vi "Test.vi"() -> ()   [LabVIEW 2017]
uses:
  Controls/saveDataOption.ctl
  TypeDefs/Trav-Command-TD.ctl
  Globals/measurementGlobal.vi
  <vilib>/Utility/file.llb/Read Delimited Spreadsheet (I64).vi
panel:
  in  "Boolean":bool
  in  "Trav Command":T1 items=["Set Reference", "Read Position", "Move", "StopMotors"]
  out "Traverse Position":i32[][](array[numeric])
  out "Block Index":i32
  in  "Setup":enum16{"Run Programme", "Show Setup"}(ring)
  in  "Data Acquisition":T2(ring)
  in  "Save Data Option":T3
  in  "Tap Control":enum32{"Plots", "Status and File"}(tab)
  out "Waveform Graph":dbl[](graph)
  out "Waveform Chart":dbl[][](graph)
  in  "Folder Path":path
  out "Comments":string
  # "ON"
  # "OFF"
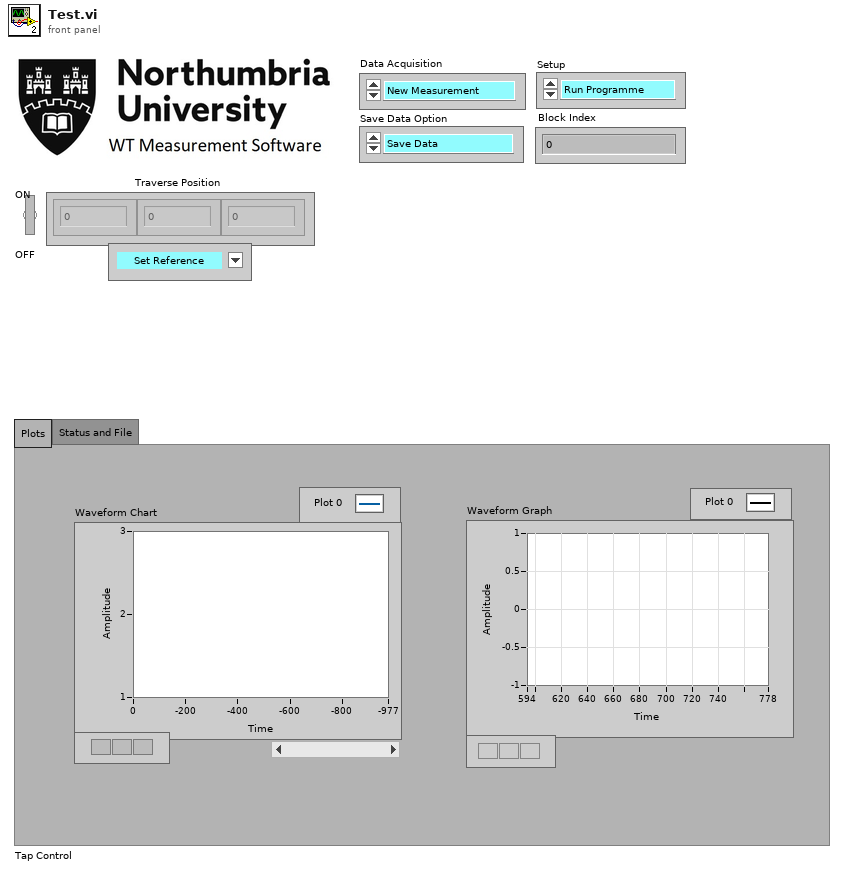
[diagram p1: front panel]
types:
  T1 = typedef "Trav-Command-TD.ctl" = u16
  T2 = enum16{"New Measurement", "Post-process Raw Data"}
  T3 = typedef "saveDataOption.ctl" = enum16{"Save Data", "Do Not Save Data"}
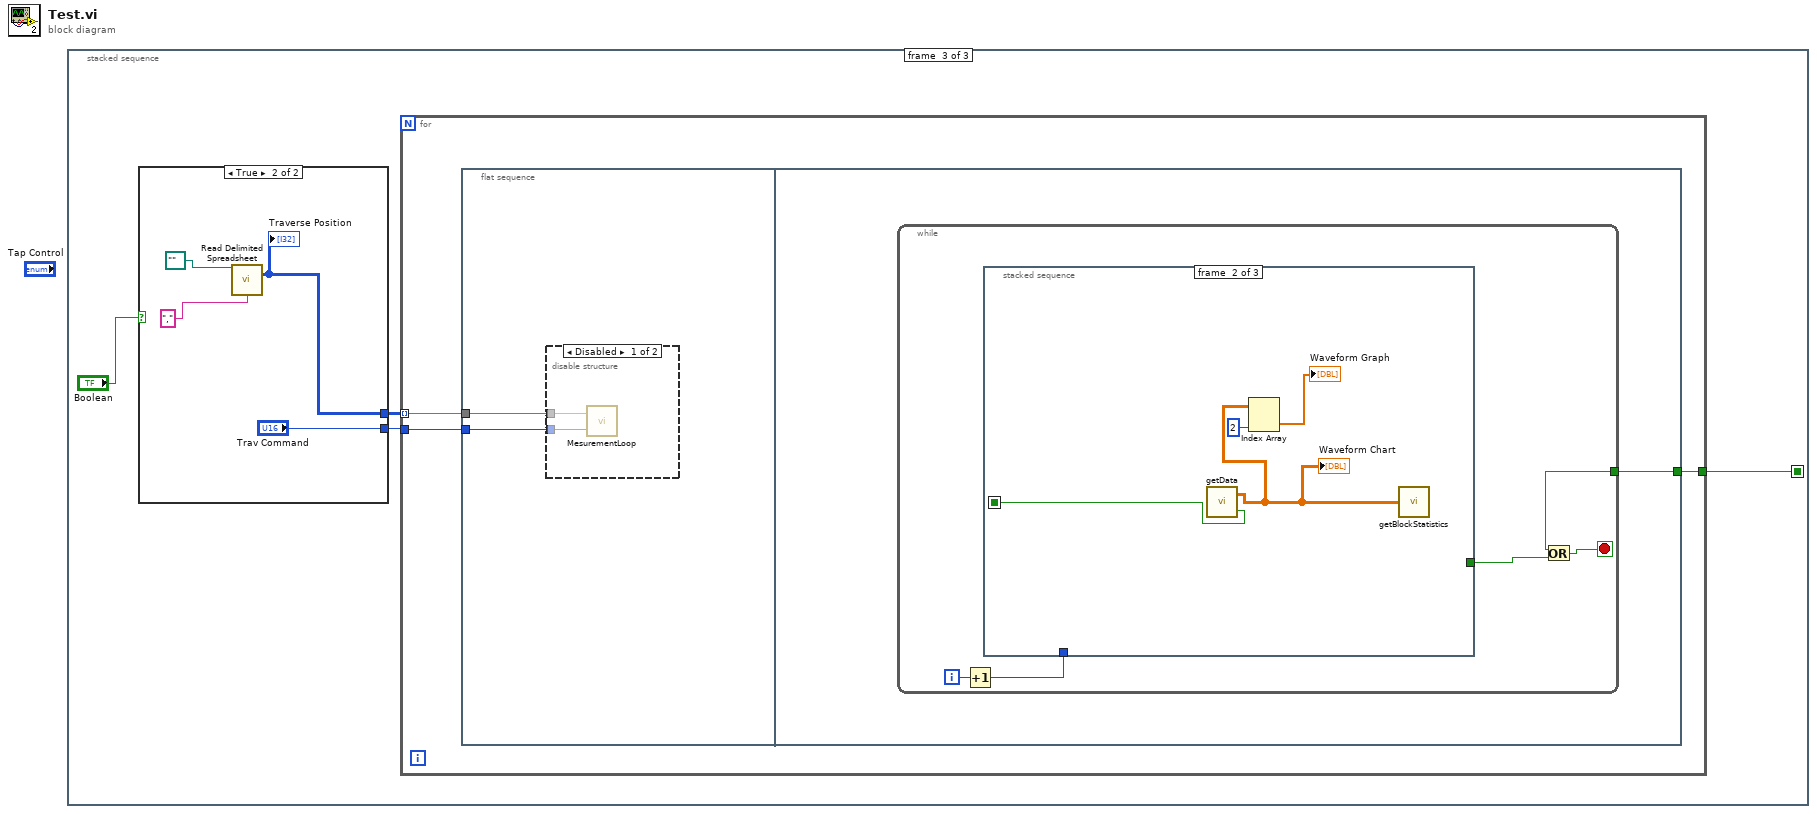
[diagram p0: block diagram]
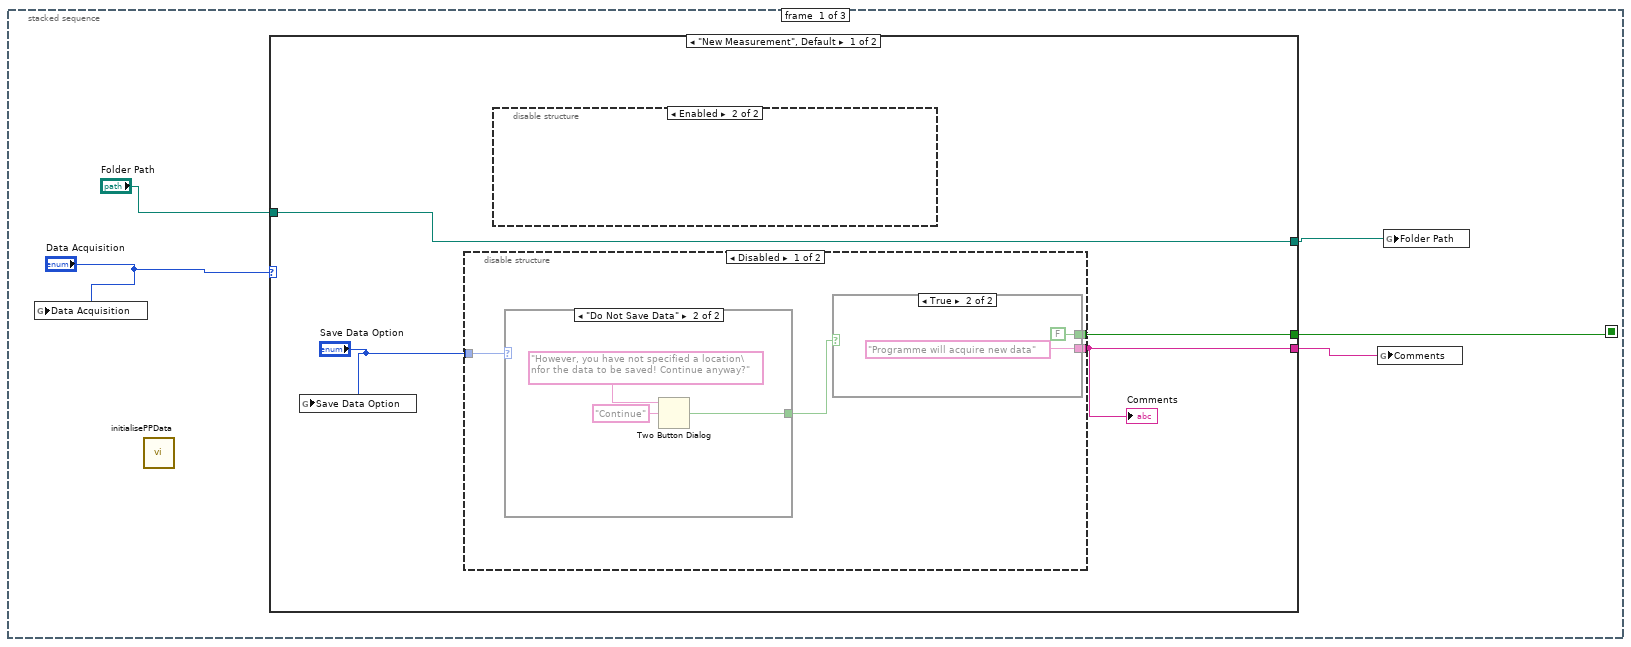
[diagram p2: hidden frame]
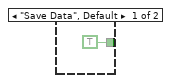
[diagram p3: hidden frame]
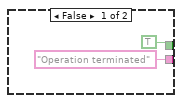
[diagram p4: hidden frame]
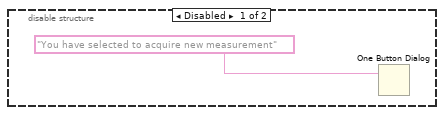
[diagram p6: hidden frame]
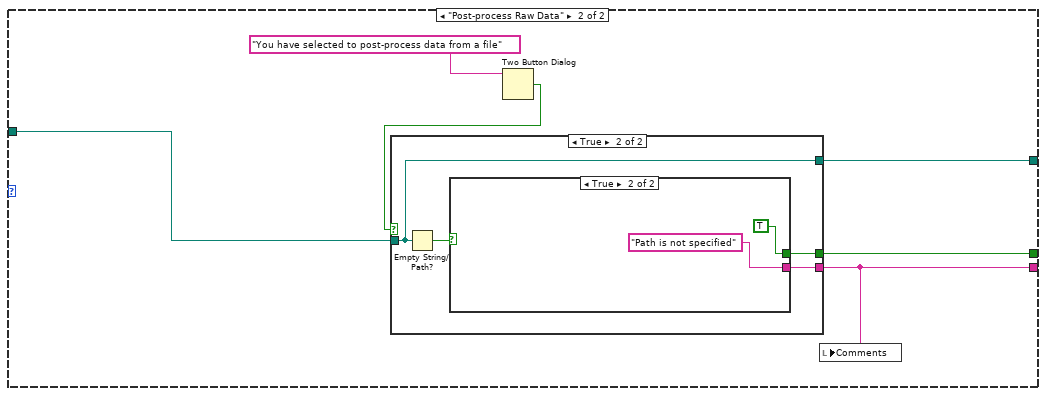
[diagram p7: hidden frame]
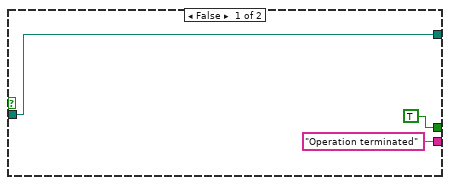
[diagram p8: hidden frame]
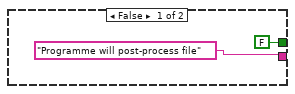
[diagram p9: hidden frame]
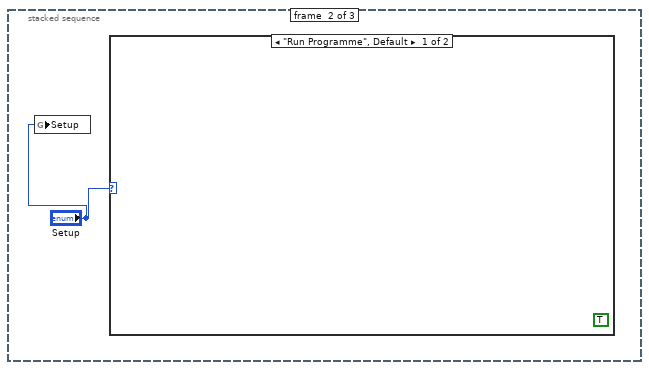
[diagram p10: hidden frame]
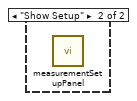
[diagram p11: hidden frame]
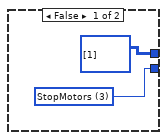
[diagram p12: hidden frame]
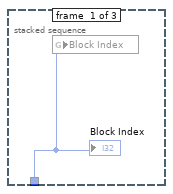
[diagram p14: hidden frame]
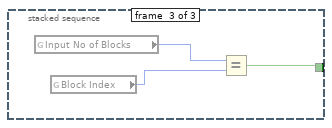
[diagram p15: hidden frame]
diagram:
  n1 = stacked-sequence {
    seq-local: [w3 _ _] -> [_ _ w44]
    frame #0 {
      n2 = global write "measurementGlobal.vi" "Data Acquisition"("Data Acquisition") -> ()
      n3 = call "initialisePPData.vi"() -> ()  [unwired: 12 in]
      n4 = case shown="\"New Measurement\", Default" "Data Acquisition" {
        tunnel: [w7 w23] -> w5
        tunnel: [w9 w24] -> w3
        tunnel: "Folder Path" -> [w8 w26]
        tunnel: [w8 w25] -> w4
        frame "New Measurement", Default {
          n5 = global write "measurementGlobal.vi" "Save Data Option"("Save Data Option") -> ()
          n6 = disable-structure shown="Disabled" {
            disable-tunnel: [w13 _] -> w9
            disable-tunnel: [w12 _] -> w7
            disable-tunnel: "Save Data Option" -> [w10 _]
            frame Disabled {
              n7 = case shown="\"Do Not Save Data\"" w10 {
                tunnel: [TRUE ("T button?") w16] -> w11
                frame "Save Data", Default {
                }
                frame "Do Not Save Data" {
                  n8 = Two Button Dialog(message="However, you have not specified a location\nfor the data to be saved! Continue anyway?", 2:"Continue" ("T button name (\"OK\")")) -> (T button?=w16:bool)  [unwired: 1 in]
                }
              }
              n9 = case shown="True" w11 {
                tunnel: ["Operation terminated" ("Comments") "Programme will acquire new data" ("Comments")] -> w12
                tunnel: [TRUE FALSE] -> w13
                frame False {
                }
                frame True {
                }
              }
            }
            frame Enabled {
            }
          }
          "Comments" <- w7
          n10 = disable-structure shown="Enabled" {
            frame Disabled {
              n11 = One Button Dialog(message="You have selected to acquire new measurement") -> ()  [unwired: 1 in, 1 out]
            }
            frame Enabled {
            }
          }
        }
        frame "Post-process Raw Data" {
          n12 = Two Button Dialog(message="You have selected to post-process data from a file") -> (T button?=w27:bool)  [unwired: 2 in]
          n13 = case shown="True" w27 {
            tunnel: w26 -> [w31 w33]
            tunnel: ["Operation terminated" w34] -> w23
            tunnel: [w31 w33] -> w25
            tunnel: [TRUE w32] -> w24
            frame False {
            }
            frame True {
              n14 = Empty String/Path?(string/path=w33) -> (empty?=w35:bool)
              n15 = case shown="True" w35 {
                tunnel: ["Programme will post-process file" "Path is not specified"] -> w34
                tunnel: [FALSE TRUE] -> w32
                frame False {
                }
                frame True {
                }
              }
            }
          }
          n16 = local write "Comments"(w23) -> ()
        }
      }
      n17 = global write "measurementGlobal.vi" "Comments"(w5) -> ()
      n18 = global write "measurementGlobal.vi" "Folder Path"(w4) -> ()
    }
    frame #1 {
      n19 = global write "measurementGlobal.vi" "Setup"("Setup") -> ()
      n20 = case shown="\"Run Programme\", Default" "Setup" {
        frame "Run Programme", Default {
          (unwired) TRUE ("Submit Setup")
        }
        frame "Show Setup" {
          n21 = call "measurementSetupPanel.vi"() -> ()  [unwired: 12 in]
        }
      }
    }
    frame #2 {
      n22 = case shown="True" "Boolean" {
        tunnel: [w46 "Trav Command"] -> w43
        tunnel: [i64[][] [[1]] ("all rows") w47] -> w42
        frame False {
          w46 = T1 3 items=["Set Reference", "Read Position", "Move", "StopMotors"] ("Trav Command")
        }
        frame True {
          n23 = call-poly <vilib>:"Read Delimited Spreadsheet.vi"("file path (dialog if empty)"=path "", "delimiter (\\t)"="," ("delimiter (\\t)")) -> ("all rows"=w47:i64[][])  [unwired: 8 in, 5 out]
          "Traverse Position" <- w47
        }
      }
      n24 = for {
        tunnel: w44 -> [w53]
        tunnel: w42 -> [w52] mode=indexing
        tunnel: w43 -> [w51]
        n25 = flat-sequence {
          tunnel: w52 -> [w55]
          tunnel: w51 -> [w54]
          tunnel: w53 -> [w58]
          frame #0 {
            n26 = disable-structure shown="Disabled" {
              disable-tunnel: w55 -> [w57 _]
              disable-tunnel: w54 -> [w56 _]
              frame Disabled {
                n27 = call "MesurementLoop.vi"("Trav Command"=w56, "All Rows"=w57) -> ()  [unwired: 1 in]
              }
              frame Enabled {
              }
            }
          }
          frame #1 {
            n28 = while {
              tunnel: w58 -> [w61]
              i -> [w63]
              stop <- w59 stop-if-true
              n29 = Increment(x=w63) -> (x+1=w62:i32)
              n30 = stacked-sequence {
                seq-local: [_ w68 _] -> [_ _ _]
                tunnel: w62 -> [w64 _ _]
                tunnel: [_ _ w69] -> w60
                frame #0 {
                  n31 = global write "measurementGlobal.vi" "Block Index"(w64) -> ()
                  "Block Index" <- w64
                }
                frame #1 {
                  n32 = call "getData.vi"() -> ("Analogue Data (volts)"=w65:dbl[][], "Error Status"=w68:bool)  [unwired: 1 in]
                  "Waveform Chart" <- w65
                  n33 = Index Array(array=w65, index (col)=2 ("disabled index (col)")) -> (element=→"Waveform Graph":dbl[])  [unwired: 1 in]
                  n34 = call "getBlockStatistics.vi"("Analogue Data (volts)"=w65) -> ()  [unwired: 1 out]
                }
                frame #2 {
                  n35 = global read "measurementGlobal.vi" "Input No of Blocks"() -> (w71:i32)
                  n36 = global read "measurementGlobal.vi" "Block Index"() -> (w70:i32)
                  n37 = Equal?(x=w71, y=w70) -> (x = y?=w69:bool)
                }
              }
              n38 = Or(x=w61, y=w60) -> (x .or. y?=w59:bool)
            }
          }
        }
      }
    }
  }
